vi "Virtualni_Osciloskop_glavni.vi"() -> ()   [LabVIEW 2014]
doc: "Example: Configured Acquisition\n\nRecommended Input Signal: 100 kHz, 4 Vpp, sine wave\n\nDevices Supported: Refer to NI Example Finder\n\nDescription:\n\nThis example configures all the digitizer's vertical, horizontal, and triggering properties before every acquisition. It allows you to experiment with numerous configurations, including acquisition types and triggering modes, since it supports nearly the entire functionality of NI-SCOPE. However, it is may be more instructive to consult other examples about specific topics such as FlexRes, Random Interleaved Sampling, and Multi-Record to learn more about these features.\n\nMany parameters are included an the front panel of this example. Notice that the \"min sample rate\" is next to the \"actual sample rate,\" and similarly the \"min record length\" is near the \"actual record length.\" The \"min\" values are specified with the Configure Horizontal Timing VI. NI-SCOPE maintains a constant time per record for each acquisition. So when you specify a min sample rate and a min record length, this determines the amount of time the acquisition should take:\n\n time per record = min record length / min sampling rate. \n\nHowever, digitizers support only a certain number of defined sampling rates, so if the value chosen is not a valid rate, it is rounded to the next higher rate, called the actual sample rate. The actual record length is then calculated in order to maintain the time per record. Both of these values are returned in this example so you can investigate the effects of parameter rounding with your digitizer. For more information about parameter coercions, see the NI High Speed Digitizers Help.\n\nThe enforce realtime property allows this example to use Random Interleaved Sampling. See the Random Interleaved Sampling example for more details.\n\nKeep in mind that not all digitizers support all the features in this example. The NI High Speed Digitizers Help includes a table of supported features for each device."
uses:
  <instrlib>/niScope/Controls/niScope vertical coupling.ctl
  <instrlib>/niScope/Controls/niScope trigger coupling.ctl
  <instrlib>/niScope/Controls/niScope trigger window mode.ctl
  <instrlib>/niScope/Controls/niScope trigger slope.ctl
  <instrlib>/niScope/Configure/Trigger/niScope Configure Trigger Edge.vi
  <instrlib>/niScope/Configure/Trigger/niScope Configure Trigger Hysteresis.vi
  <instrlib>/niScope/Configure/Trigger/niScope Configure Trigger Digital.vi
  <instrlib>/niScope/Configure/Trigger/niScope Configure Trigger Window.vi
  <instrlib>/niScope/Configure/Trigger/niScope Configure Trigger Immediate.vi
  <instrlib>/niScope/Acquire/Fetch/niScope Multi Fetch Cluster.vi
  <vilib>/measure/maspectr.llb/FFT Power Spectrum and PSD for 1 Chan.vi
  <vilib>/measure/mascope.llb/Amplitude and Levels 1 chan.vi
  <vilib>/measure/NI_MAPro.lvlib
panel:
  out "Power Spectrum / PSD":cluster{"f0":dbl, "df":dbl, "magnitude":dbl[]} {"magnitude" format="%.2p"; "f0" format="%0.2p"; "df" format="%0.2p"}
  out "Vpp":dbl
  out "low state level":dbl format="%.2g"
  out "high state level":dbl format="%.2g"
  out "amplitude":dbl format="%.2p"
  out "auto triggered":bool caption="Auto Triggered"
  in  "trigger modifier":i32(ring)=1 caption="Trigger Modifier" items=["None"=1, "Auto Trigger"=2]
  in  "Enable TIS":bool
  in  "trigger source":string(combo)="0" caption="Trigger Source"
  in  "trigger slope":T1 caption="Trigger Slope"
  in  "trigger window mode":T2 caption="Window Mode"
  in  "trigger coupling":T3=1 caption="Trigger Coupling" items=["AC"=0, "DC"=1, "HF Reject"=3, "LF Reject"=4, "AC Plus HF Reject"=1001]
  in  "vertical coupling":T4=1 caption="Vertical Coupling" items=["AC", "DC", "Ground"]
  out "error out":errorcluster {"code" format="%.0x"}
  in  "stop":bool
  in  "high level":dbl=0.1 caption="Window High Level" format="%.2f"
  in  "low level":dbl=-0.1 caption="Window Low Level" format="%.2f"
  in  "hysteresis":dbl=0.05 caption="Hysteresis" format="%.2f"
  in  "trigger level":dbl caption="Trigger Level" format="%.2f"
  in  "reference position":dbl=50.0 caption="Ref Position" format="%.1f"
  in  "trigger delay":dbl caption="Trigger Delay" format="%.4p"
  in  "maximum input frequency":dbl caption="Max. Input Frequency" format="%.2f"
  in  "input impedance":u32(ring) caption="Input Impedance" items=["1 mega ohm"=0, "50 ohms"=2]
  in  "probe attenuation":dbl=1.0 caption="Probe Attenuation" format="%.1f"
  in  "vertical offset":dbl caption="Vertical Offset" format="%.4f"
  in  "timeout (s)":dbl=5.0 caption="Timeout(s)" format="%.2f"
  in  "trigger type":T5(ring)=enum."Immediate" caption="Trigger Type"
  out "actual sample rate":dbl=10000000.0 caption="Actual Sample Rate" format="%.2p"
  out "actual record length":i32=1000 caption="Actual Record Length"
  out "Waveform Graph":T6(graph)
  in  "min record length":i32=1000 caption="Min. Record Length"
  in  "min sample rate":dbl=10000000.0 caption="Min. Sample Rate" step=1000000.0 format="%.2p"
  in  "vertical range":dbl=10.0 caption="Vertical Range (V)" format="%.2f"
  in  "enforce realtime":bool=TRUE caption="Enforce Realtime"
  in  "channel name":string="0" caption="Channel Name(s)"
  in  "resource name":refnum<k15>="DAQ::1" caption="Resource Name"
  # "Vertical"
  # "Channel"
  # "Trigger"
  # "Specific Parameters - Not all parameters \napply to all trigger types."
  # "Trigger Selection"
  # "Horizontal"
  # "Common Parameters"
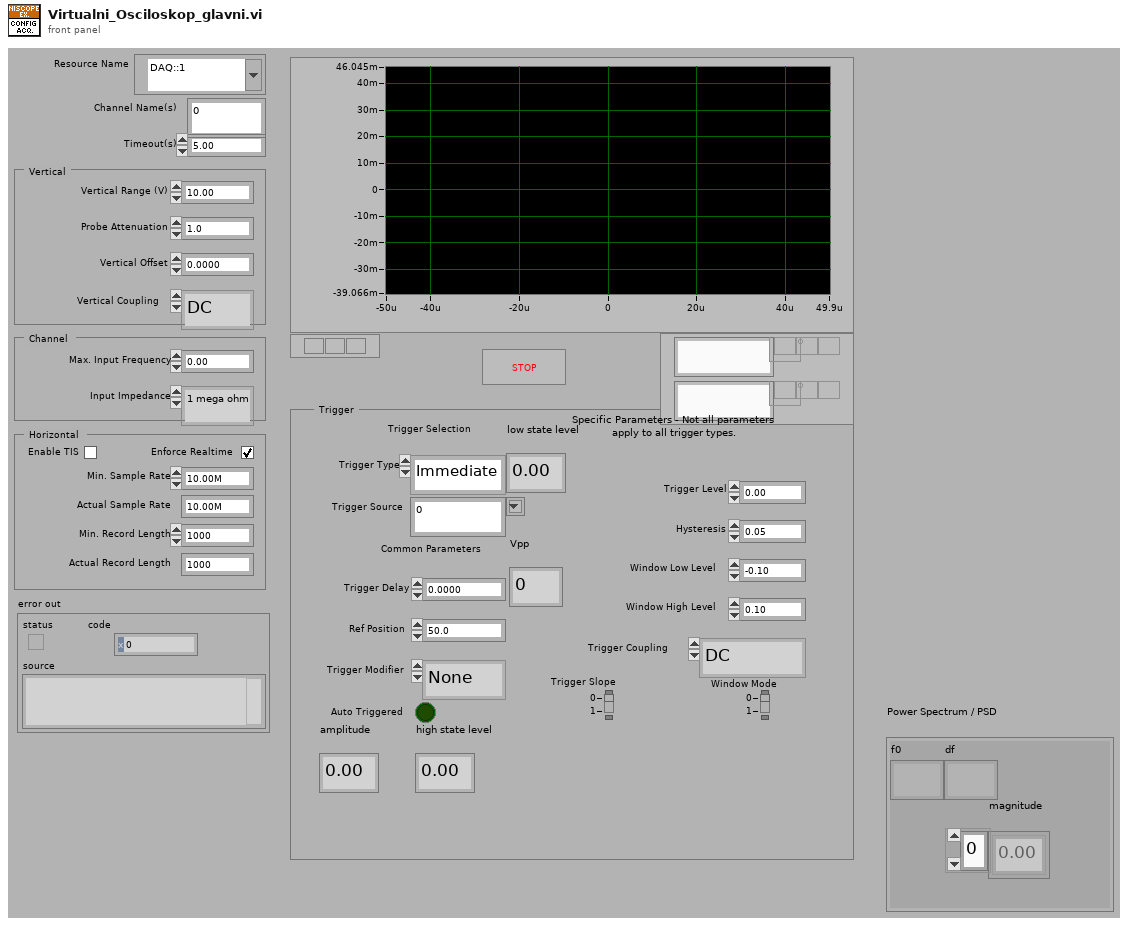
[diagram p1: front panel]
types:
  T1 = typedef "niScope trigger slope.ctl" = i32
  T2 = typedef "niScope trigger window mode.ctl" = i32
  T3 = typedef "niScope trigger coupling.ctl" = u16
  T4 = typedef "niScope vertical coupling.ctl" = i32
  T5 = enum16{"Edge", "Hysteresis", "Digital", "Window", "Immediate"}
  T6 = cluster{"relativeInitialX":dbl, "xIncrement":dbl, "wfm":dbl[]}[]
  T7 = cluster{"relativeInitialX":dbl, "xIncrement":dbl, "wfm":dbl[]}
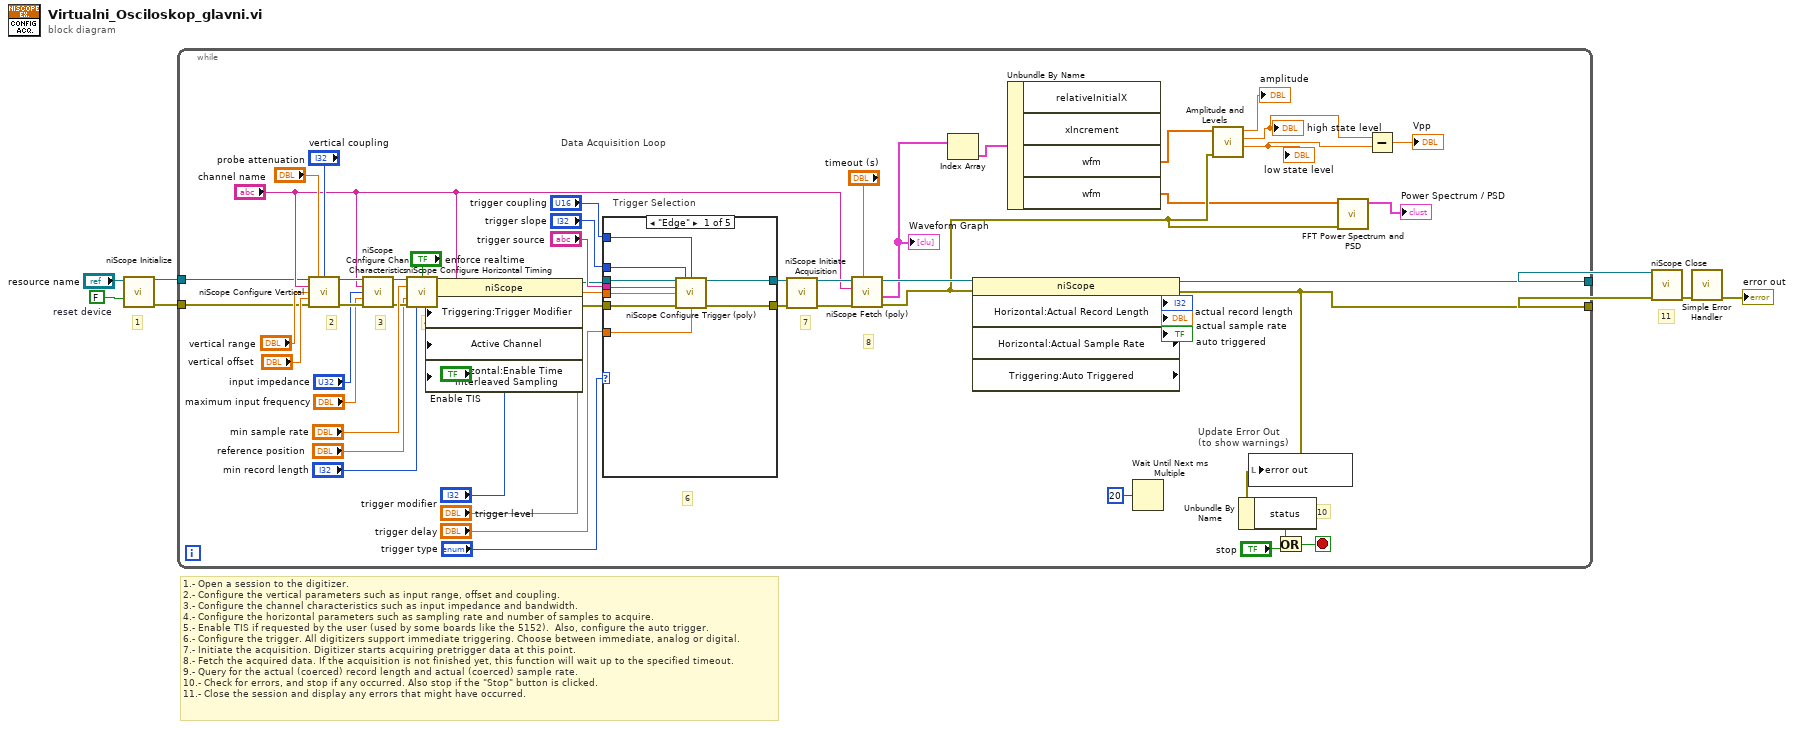
[diagram p0: block diagram]
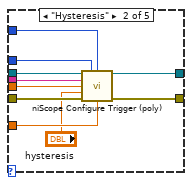
[diagram p2: hidden frame]
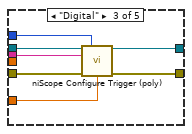
[diagram p3: hidden frame]
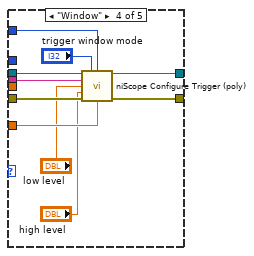
[diagram p4: hidden frame]
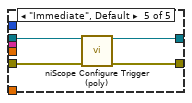
[diagram p5: hidden frame]
diagram:
  w8 = FALSE  # reset device
  # "11"
  # "1.- Open a session to the digitizer.\n2.- Configure the vertical parameters such as input range, offset and coupling.\n3.- Configure the channel characteristics such as input impedance and bandwidth.\n4.- Configure the horizontal parameters such as sampling rate and number of samples to acquire.\n5.- Enable TIS if requested by the user (used by some boards like the 5152).  Also, configure the auto trigger.\n6.- Configure the trigger. All digitizers support immediate triggering. Choose between immediate, analog or digital.\n7.- Initiate the acquisition. Digitizer starts acquiring pretrigger data at this point.\n8.- Fetch the acquired data. If the acquisition is not finished yet, this function will wait up to the specified timeout.\n9.- Query for the actual (coerced) record length and actual (coerced) sample rate.\n10.- Check for errors, and stop if any occurred. Also stop if the \"Stop\" button is clicked.\n11.- Close the session and display any errors that might have occurred."
  # "1"
  n1 = call <instrlib>:"niScope Initialize.vi"("resource name"="resource name", "reset device"=w8) -> ("instrument handle"=w1:refnum<k15>, "error out"=w4:errorcluster)  [unwired: 12 in]
  n2 = while {
    tunnel: w4 -> [w25]
    tunnel: [w20] -> w3
    tunnel: [w23] -> w2
    tunnel: w1 -> [w26]
    stop <- w45 stop-if-true
    # "5"
    # "2"
    # "3"
    # "4"
    # "6"
    # "7"
    # "8"
    # "9"
    # "10"
    # "Update Error Out\n(to show warnings)"
    # "Data Acquisition Loop"
    n3 = call <instrlib>:"niScope Configure Vertical.vi"("instrument handle"=w26, "probe attenuation"="probe attenuation", "vertical coupling"="vertical coupling", "channels"="channel name", "vertical range"="vertical range", "vertical offset"="vertical offset", "error in"=w25) -> ("instrument handle out"=w59:refnum<k15>, "error out"=w58:errorcluster)  [unwired: 7 in]
    n4 = call <instrlib>:"niScope Configure Chan Characteristics.vi"("instrument handle"=w59, "channels"="channel name", "input impedance"="input impedance", "maximum input frequency"="maximum input frequency", "error in"=w58) -> ("instrument handle out"=w56:refnum<k15>, "error out"=w57:errorcluster)  [unwired: 9 in]
    n5 = call <instrlib>:"niScope Configure Horizontal Timing.vi"("instrument handle"=w56, "enforce realtime"="enforce realtime", "min sample rate"="min sample rate", "reference position"="reference position", "error in"=w57, "min record length"="min record length") -> ("instrument handle out"=w34:refnum<k15>, "error out"=w33:errorcluster)  [unwired: 8 in]
    n6 = property class="niScope"(reference=w34, error in=w33, "Triggering:Trigger Modifier"="trigger modifier", "Active Channel"="channel name", "Horizontal:Enable Time Interleaved Sampling"="Enable TIS") -> (reference out=w31:refnum<k15>, error out=w32:errorcluster)
    n7 = case "Trigger Selection" shown="\"Edge\"" "trigger type" {
      tunnel: w32 -> [w71 w81 w88 w98 w102]
      tunnel: [w66 w76 w83 w93 w99] -> w41
      tunnel: w31 -> [w70 w80 w87 w97 w101]
      tunnel: [w67 w78 w84 w94 w100] -> w44
      tunnel: "trigger source" -> [w69 w79 w86 w96 _]
      tunnel: "trigger delay" -> [w68 w77 w85 w95 _]
      tunnel: "trigger level" -> [w65 w73 _ _ _]
      tunnel: "trigger slope" -> [w64 w75 w82 _ _]
      tunnel: "trigger coupling" -> [w63 w74 _ w92 _]
      frame "Edge" {
        n8 = call-poly <instrlib>:"niScope Configure Trigger (poly).vi"("instrument handle"=w70, "trigger slope"=w64, "trigger coupling"=w63, "trigger source"=w69, "trigger level"=w65, "error in"=w71, "trigger delay"=w68) -> ("instrument handle out"=w67:refnum<k15>, "error out"=w66:errorcluster)  [unwired: 7 in]
      }
      frame "Hysteresis" {
        n9 = call-poly <instrlib>:"niScope Configure Trigger (poly).vi"("instrument handle"=w80, "trigger slope"=w75, "trigger coupling"=w74, "trigger source"=w79, "trigger level"=w73, "hysteresis"="hysteresis", "error in"=w81, "trigger delay"=w77) -> ("instrument handle out"=w78:refnum<k15>, "error out"=w76:errorcluster)  [unwired: 6 in]
      }
      frame "Digital" {
        n10 = call-poly <instrlib>:"niScope Configure Trigger (poly).vi"("instrument handle"=w87, "trigger slope"=w82, "trigger source"=w86, "error in"=w88, "trigger delay"=w85) -> ("instrument handle out"=w84:refnum<k15>, "error out"=w83:errorcluster)  [unwired: 9 in]
      }
      frame "Window" {
        n11 = call-poly <instrlib>:"niScope Configure Trigger (poly).vi"("instrument handle"=w97, "trigger window mode"="trigger window mode", "trigger coupling"=w92, "trigger source"=w96, "low level"="low level", "high level"="high level", "error in"=w98, "trigger delay"=w95) -> ("instrument handle out"=w94:refnum<k15>, "error out"=w93:errorcluster)  [unwired: 6 in]
      }
      frame "Immediate", Default {
        n12 = call-poly <instrlib>:"niScope Configure Trigger (poly).vi"("instrument handle"=w101, "error in"=w102) -> ("instrument handle out"=w100:refnum<k15>, "error out"=w99:errorcluster)  [unwired: 12 in]
      }
    }
    n13 = call <instrlib>:"niScope Initiate Acquisition.vi"("instrument handle"=w44, "error in"=w41) -> ("instrument handle out"=w43:refnum<k15>, "error out"=w42:errorcluster)  [unwired: 12 in]
    n14 = call-poly <instrlib>:"niScope Fetch (poly).vi"("timeout"="timeout (s)", "error in"=w42, "channels"="channel name", "instrument handle"=w43) -> ("error out"=w11:errorcluster, "waveform"=w18:T6, "instrument handle out"=w24:refnum<k15>)  [unwired: 4 in, 1 out]
    "Waveform Graph" <- w18
    n15 = Index Array(array=w18) -> (element=w17:T7)  [unwired: 1 in]
    n16 = property class="niScope"(reference=w24, error in=w11) -> (reference out=w23:refnum<k15>, error out=w20:errorcluster, "Horizontal:Actual Record Length"=→"actual record length":i32, "Horizontal:Actual Sample Rate"=→"actual sample rate":dbl, "Triggering:Auto Triggered"=→"auto triggered":bool)
    n17 = Unbundle By Name(w17) -> ("wfm"=w16:dbl[], "wfm"=w10:dbl[])  [unwired: 2 out]
    n18 = Wait Until Next ms Multiple(millisecond multiple=u32 20 ("milliseconds to wait")) -> ()  [unwired: 1 out]
    n19 = call-poly <vilib>:"Amplitude and Levels.vi"("error in (no error)"=w11, "signal in"=w16) -> ("low state level"=w14:dbl, "high state level"=w13:dbl, "amplitude"=→"amplitude":dbl)  [unwired: 6 in, 1 out]
    "high state level" <- w13
    "low state level" <- w14
    n20 = Unbundle By Name(w20) -> ("status"=w40:bool)
    n21 = local write "error out"(w20) -> ()
    n22 = Or(x=w40, y="stop") -> (x .or. y?=w45:bool)
    n23 = call-poly <vilib>:"FFT Power Spectrum and PSD.vi"("error in (no error)"=w11, "time signal"=w10) -> ("Power Spectrum / PSD"=→"Power Spectrum / PSD":cluster{"f0":dbl, "df":dbl, "magnitude":dbl[]})  [unwired: 6 in, 3 out]
    n24 = Subtract(x=w13, y=w14) -> (x-y=→"Vpp":dbl)
  }
  n25 = call <instrlib>:"niScope Close.vi"("instrument handle"=w2, "error in"=w3) -> ("error out"=w6:errorcluster)  [unwired: 13 in]
  n26 = call <vilib>:"Simple Error Handler.vi"("error in (no error)"=w6) -> ("error out"=→"error out":errorcluster)  [unwired: 4 in, 4 out]
